vi "Constructor.vi"(8 "ErrorIn":errorcluster, 11 "TemplateGUITAFIn":refnum<class "TemplateGUITAF.lvclass">) -> (0 "ErrorOut":errorcluster, 3 "TemplateGUITAFOut":refnum<class "TemplateGUITAF.lvclass">)   [LabVIEW 2021, in "TemplateGUITAF.lvlib" / "TemplateGUITAF.lvclass"]
uses:
  TemplateGUITAF.lvclass
  TemplateGUITAF.lvclass/TemplateGUITAF.ctl
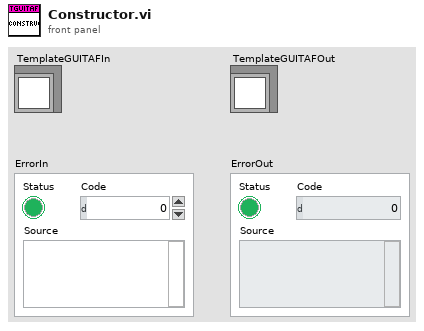
[diagram p1: front panel]
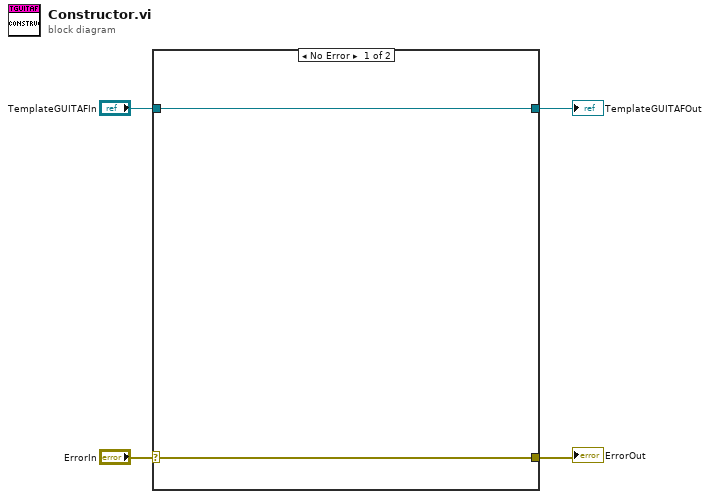
[diagram p0: block diagram]
diagram:
  n1 = case shown="No Error" "ErrorIn" {
    selector: "ErrorIn" -> [w5 w8]
    tunnel: [w5 w8] -> w3
    tunnel: [w6 w7] -> w1
    tunnel: "TemplateGUITAFIn" -> [w6 w7]
    frame No Error {
    }
    frame Error {
    }
  }
  "ErrorOut" <- w3
  "TemplateGUITAFOut" <- w1
